vi "LoadClassFromName_core.vi"(7 "ClassTemplate":refnum<class>, 8 "error in (no error)":errorcluster, 9 "AdditionalData":variant, 10 "Class":string, 11 "DLMapper in":refnum<class "ClassLoader_lib.lvclass">) -> (0 "error out":errorcluster, 2 "Class":refnum<class>, 3 "DLMapper out":refnum<class "ClassLoader_lib.lvclass">)   [LabVIEW 2020, in "ClassLoader.lvlib" / "ClassLoader_lib.lvclass"]
uses:
  ClassLoader_lib.lvclass
  ClassLoader/ClassLoader.lvclass
  <vilib>/Utility/LVLibp/NI_PackedLibraryUtility.lvlib
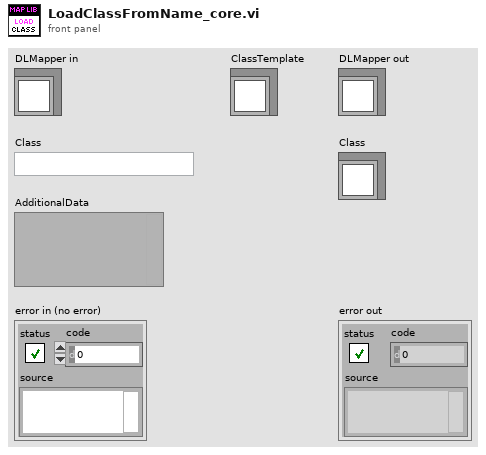
[diagram p1: front panel]
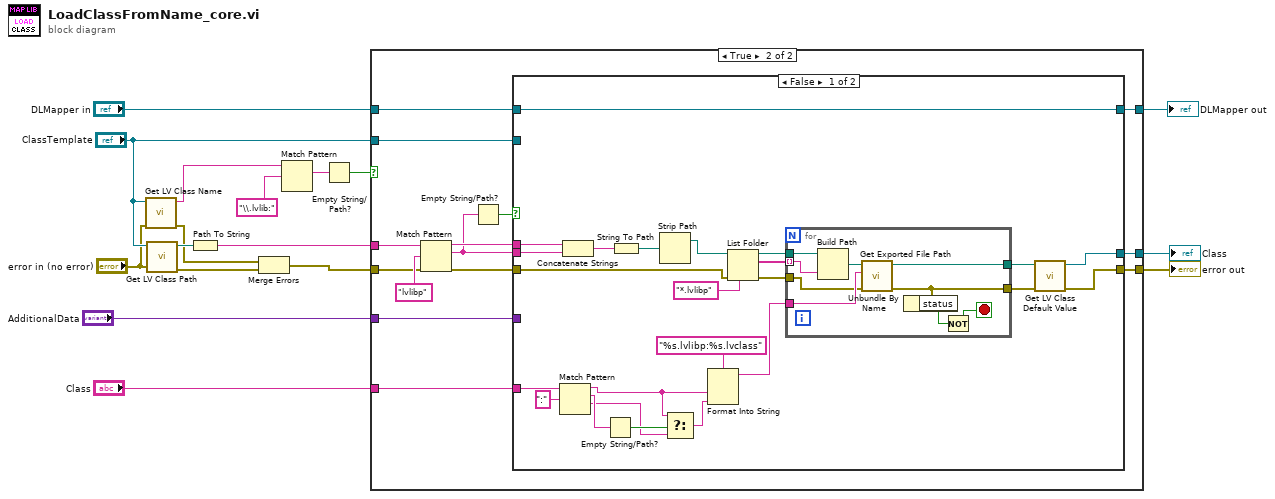
[diagram p0: block diagram]
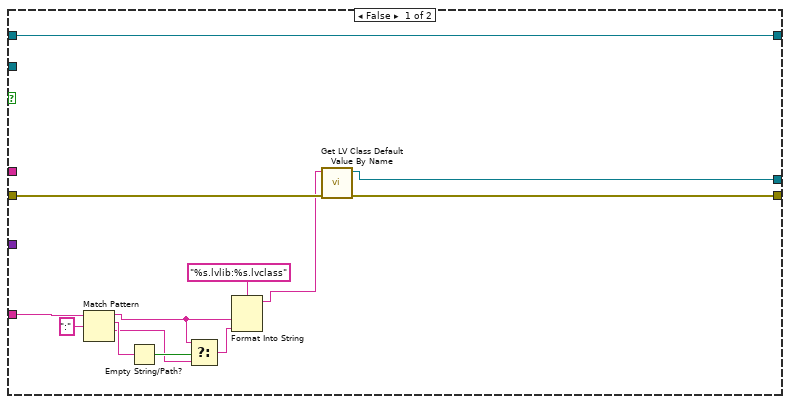
[diagram p2: hidden frame]
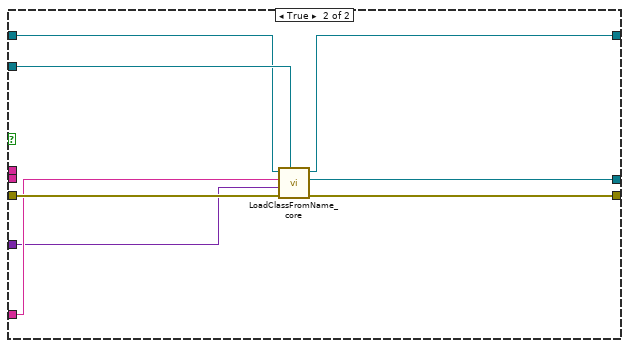
[diagram p3: hidden frame]
diagram:
  n1 = call <vilib>:"Get LV Class Name.vi"("error in (no error)"="error in (no error)", "object"="ClassTemplate") -> ("error out"=w2:errorcluster, "class name"=w1:string)  [unwired: 8 in]
  n2 = call <vilib>:"Get LV Class Path.vi"("error in (no error)"="error in (no error)", "object"="ClassTemplate") -> ("error out"=w16:errorcluster, "class path"=w17:path)  [unwired: 8 in]
  n3 = Path To String(path=w17) -> (string=w11:string)
  n4 = Merge Errors(w2, w16) -> (w3:errorcluster)
  n5 = Match Pattern(string=w1, regular expression="\\.lvlib:") -> (match substring=w10:string)  [unwired: 1 in, 3 out]
  n6 = Empty String/Path?(string/path=w10) -> (empty?=w9:bool)
  n7 = case shown="True" w9 {
    tunnel: w3 -> [w21 w41]
    tunnel: [w18 w40] -> w15
    tunnel: [w19 w39] -> w14
    tunnel: "Class" -> [w23 w38]
    tunnel: w11 -> [_ w37]
    tunnel: "AdditionalData" -> [_ w34]
    tunnel: "ClassTemplate" -> [_ w33]
    tunnel: "DLMapper in" -> [w30 w32]
    tunnel: [w30 w31] -> w6
    frame False {
      n8 = Match Pattern(string=w23, regular expression=":") -> (before substring=w25:string, match substring=w28:string, after substring=w26:string)  [unwired: 1 in, 1 out]
      n9 = Empty String/Path?(string/path=w28) -> (empty?=w27:bool)
      n10 = Select(t=w25, s=w27, f=w26) -> (s? t:f=w24:string)
      n11 = Format Into String(format string="%s.lvlib:%s.lvclass", w25, w24) -> (resulting string=w20:string)  [unwired: 2 in, 1 out]
      n12 = call <vilib>:"Get LV Class Default Value By Name.vi"("error in (no error)"=w21, "class name"=w20) -> ("error out"=w18:errorcluster, "object"=w19:refnum<class>)  [unwired: 8 in]
    }
    frame True {
      n13 = Match Pattern(string=w37, regular expression="lvlibp") -> (before substring=w42:string, match substring=w36:string)  [unwired: 1 in, 2 out]
      n14 = Empty String/Path?(string/path=w36) -> (empty?=w35:bool)
      n15 = case shown="False" w35 {
        tunnel: w42 -> [w67 _]
        tunnel: w41 -> [w57 w84]
        tunnel: [w48 w83] -> w40
        tunnel: [w47 w82] -> w39
        tunnel: w38 -> [w46 w81]
        tunnel: w36 -> [w45 _]
        tunnel: w34 -> [_ w80]
        tunnel: w33 -> [_ w79]
        tunnel: w32 -> [w44 w78]
        tunnel: [w44 w77] -> w31
        frame False {
          n16 = Match Pattern(string=w46, regular expression=":") -> (before substring=w52:string, match substring=w55:string, after substring=w53:string)  [unwired: 1 in, 1 out]
          n17 = Concatenate Strings(w67, w45) -> (w66:string)
          n18 = Empty String/Path?(string/path=w55) -> (empty?=w54:bool)
          n19 = String To Path(string=w66) -> (path=w65:path)
          n20 = Strip Path(path=w65) -> (stripped path=w64:path)  [unwired: 1 out]
          n21 = Select(t=w52, s=w54, f=w53) -> (s? t:f=w51:string)
          n22 = Format Into String(format string="%s.lvlibp:%s.lvclass", w52, w51) -> (resulting string=w58:string)  [unwired: 2 in, 1 out]
          n23 = List Folder(path=w64, pattern="*.lvlibp", error in=w57) -> (path out=w62:path, filenames=w61:string[], error out=w56:errorcluster)  [unwired: 1 in, 1 out]
          n24 = for {
            tunnel: w62 -> [w76]
            tunnel: w61 -> [w75] mode=indexing
            tunnel: [w71] -> w50
            tunnel: w58 -> [w73]
            tunnel: w56 -> [w72]
            tunnel: [w68] -> w49
            stop <- w69 stop-if-true
            n25 = Build Path(base path=w76, name or relative path=w75) -> (appended path=w74:path)
            n26 = call <vilib>:"Get Exported File Path.vi"("error in (no error)"=w72, "qualified name"=w73, "packed library path"=w74) -> ("error out"=w71:errorcluster, "path"=w68:path)  [unwired: 7 in]
            n27 = Unbundle By Name(w71) -> ("status"=w70:bool)
            n28 = Not(x=w70) -> (.not. x?=w69:bool)
          }
          n29 = call <vilib>:"Get LV Class Default Value.vi"("error in (no error)"=w50, "class path"=w49) -> ("error out"=w48:errorcluster, "object"=w47:refnum<class>)  [unwired: 8 in]
        }
        frame True {
          n30 = call-parent "LoadClassFromName_core.vi"("ClassTemplate"=w79, "error in (no error)"=w84, "AdditionalData"=w80, "Class"=w81, "DLMapper in"=w78) -> ("error out"=w83:errorcluster, "Class"=w82:refnum<class>, "DLMapper out"=w77:refnum<class "ClassLoader_lib.lvclass">)  [unwired: 4 in]
        }
      }
    }
  }
  "error out" <- w15
  "DLMapper out" <- w6
  "Class" <- w14
